vi "Main.vi"   [LabVIEW 2017]
uses:
  <vilib>/Platform/TimedLoop/XDataNode/timing_clust.ctl
  <vilib>/Platform/TimedLoop/XDataNode/nitl_modes.ctl
  <vilib>/Platform/TimedLoop/XDataNode/wakeup.ctl
  Controls/State.ctl
  <vilib>/platform/TimedLoop/XDataNode/XDataNode.xnode
  <vilib>/Platform/TimedLoop/XDataNode/XDNodeRunTimeDep.lvlib
types:
  T1 = typedef "State.ctl" = enum16{"Standby", "Initialize", "Pusher", "Live", "Norm Brake", "E-Stop"}
  T2 = typedef "XDNodeRunTimeDep.lvlib/timing_clust.ctl" = cluster{"Expected End [f-1]":u64, "Actual End [f-1]":u64, "Finished Late? [f-1]":bool, "Expected End [i-1]":u64, "Actual End [i-1]":u64, "Finished Late? [i-1]":bool, "Expected Start [i]":u64, "Actual Start [i]":u64, "Expected Start [f]":u64, "Actual Start [f]":u64, "Source Name":string, "Structure Name":string, "Period":i64, "Deadline":i64, "Offset":i64, "Start":i64, "Priority":i32, "Timeout":i32, "Mode":T3, "Wakeup Reason":T4, "Error":errorcluster, "Source Type":string, "Secondary Source Type":string, "Global End Time":u64, "Global Start Time":u64, "Frame Duration":u64, "Iteration Duration":u64, "Assigned CPU":i32, "I/O Scan Engine Mode":u32}
  T3 = typedef "XDNodeRunTimeDep.lvlib/nitl_modes.ctl" = enum32{"No Change", "Process missed periods, maintain original phase", "Discard missed periods, maintain original phase", "Process missed periods, ignore original phase", "Discard missed periods, ignore original phase"}
  T4 = typedef "XDNodeRunTimeDep.lvlib/wakeup.ctl" = enum32{"Normal", "Aborted", "Asynchronous wakeup", "Timing source error", "Timed loop error", "Timeout"}
  T5 = cluster{"X dtheta":sgl, "Y dtheta":sgl, "Z dtheta":sgl, "X accel":sgl, "Y accel":sgl, "Z accel":sgl, "Velocity":sgl, "IMU Fault":bool, "Time Since Last Tape":sgl, "Position":sgl}
  T6 = cluster{"Primary Battery 1 Voltage":sgl, "Primary Battery 2 Voltage":sgl, "Reserve Battery Voltage":sgl, "Primary Battery 1 Current":sgl, "Primary Battery 2 Current":sgl, "Reserve Battery Current":sgl, "Primary Battery 1 Temperature":sgl, "Primary Battery 2 Temperature":sgl, "Reserve Battery Temperature":sgl, "Primary Battery 1 Low":bool, "Primary Battery 2 Low":bool, "Reserve Battery Low":bool, "Primary Battery 1 Critical":bool, "Primary Battery 2 Critical":bool, "Reserve Battery Critical":bool, "Primary Battery 1 Hot":bool, "Primary Battery 2 Hot":bool, "Reserve Battery Hot":bool, "Frame Temperature":sgl, "Frame Hot":bool, "Ambient Pressure":sgl, "Tank Pressure":sgl, "Downstream Pressure":sgl, "Tank Pressue Low":bool, "Downstream Pressure Low":bool, "Tank Pressure Fault":bool, "Downstream Pressure Fault":bool, "IR 1 RAW":sgl, "IR 2 RAW":sgl, "IR Fault":bool, "Pusher Connected":bool, "Left Tape Count":u32, "Right Tape Count":u32, "Left Velocity":sgl, "Right Velocity":sgl, "Left LS Fault":bool, "Right LS Fault":bool, "Levitation Height":sgl, "Levitating?":bool, "PCS 1 Position":sgl, "PCS 2 Position":sgl, "PCS 3 Position":sgl, "PCS 4 Position":sgl, "FL Count":u8, "FR Count":u8, " BL Count":u8, "BR Count":u8}
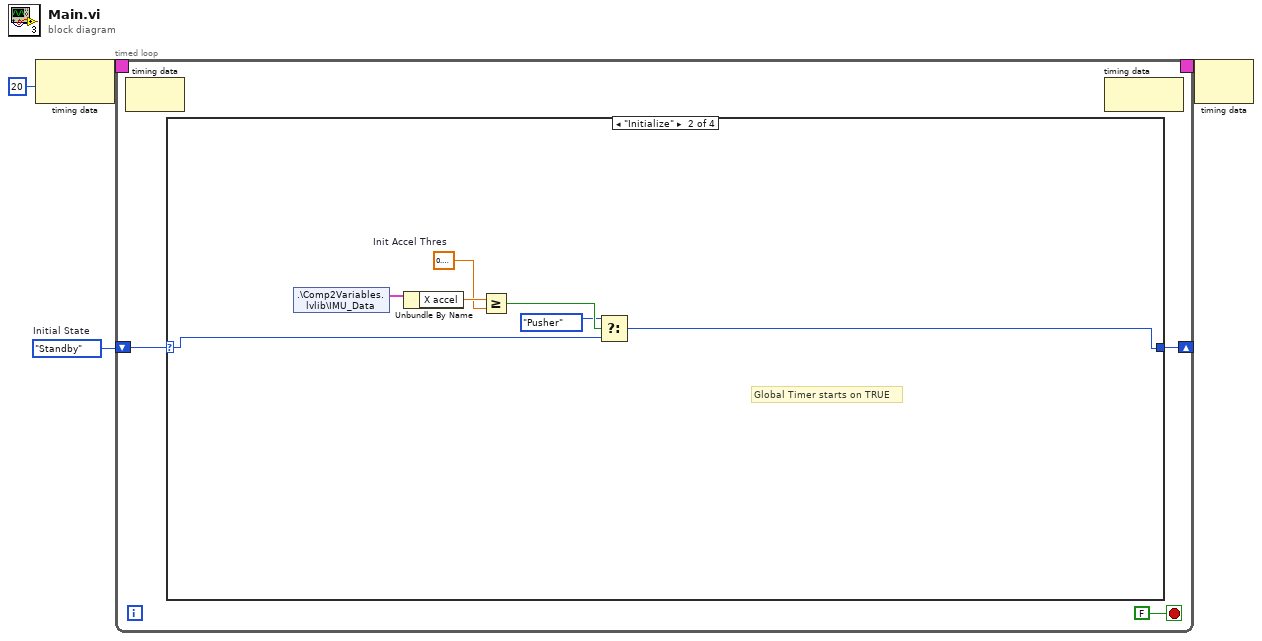
[diagram p0: block diagram]
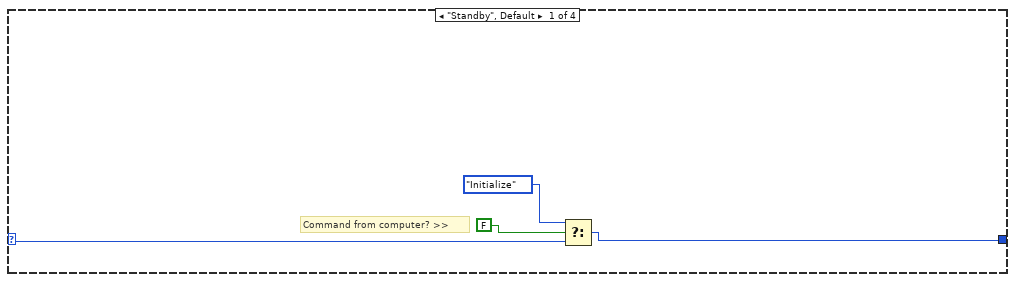
[diagram p2: hidden frame]
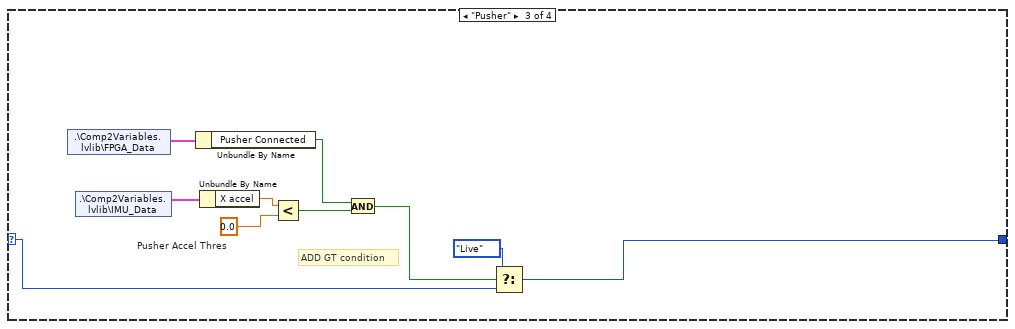
[diagram p3: hidden frame]
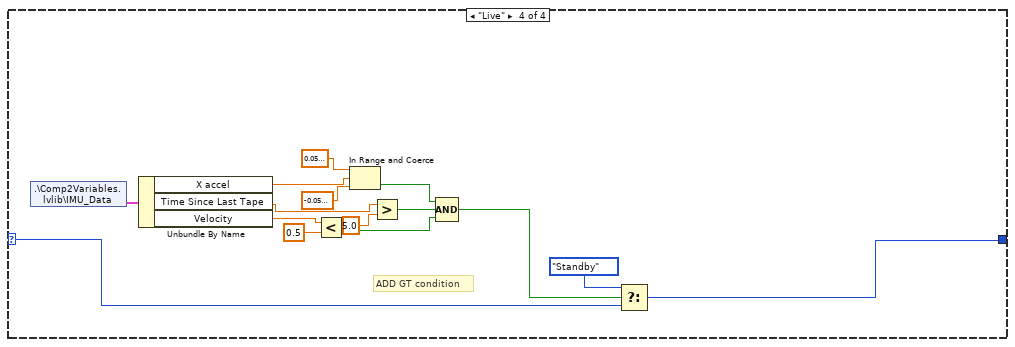
[diagram p4: hidden frame]
diagram:
  w1 = State."Standby"  # Initial State
  n1 = node-c288(i64 20 ("Period")) -> (w4:T2)
  n2 = timed-loop {
    timing: w4 -> [_]
    timing-out: [_] -> w3
    shift-right: [w5] -> _
    shift-left: w1 -> [w6]
    stop <- FALSE stop-if-true
    n3 = node-c288() -> ()  [unwired: 1 in, 1 out]
    n4 = case shown="\"Initialize\"" w6 {
      selector: w6 -> [w10 w13 w22 w31]
      tunnel: [w11 w12 w19 w30] -> w5
      frame "Standby", Default {
        # "Command from computer? >>"
        n5 = Select(t=State."Initialize" ("Initial State"), s=FALSE, f=w10) -> (s? t:f=w11:T1)
      }
      frame "Initialize" {
        w16 = sgl 0.2  # Init Accel Thres
        # "Global Timer starts on TRUE"
        n6 = shared-variable ".\\Comp2Variables.lvlib\\IMU_Data"() -> (w18:T5)  [unwired: 1 in, 1 out]
        n7 = Unbundle By Name(w18) -> ("X accel"=w17:sgl)
        n8 = Greater Or Equal?(x=w17, y=w16) -> (x >= y?=w15:bool)
        n9 = Select(t=State."Pusher", s=w15, f=w13) -> (s? t:f=w12:T1)
      }
      frame "Pusher" {
        w26 = sgl 0.0  # Pusher Accel Thres
        # "ADD GT condition"
        n10 = shared-variable ".\\Comp2Variables.lvlib\\FPGA_Data"() -> (w25:T6)  [unwired: 1 in, 1 out]
        n11 = shared-variable ".\\Comp2Variables.lvlib\\IMU_Data"() -> (w28:T5)  [unwired: 1 in, 1 out]
        n12 = Unbundle By Name(w25) -> ("Pusher Connected"=w24:bool)
        n13 = Unbundle By Name(w28) -> ("X accel"=w27:sgl)
        n14 = Less?(x=w27, y=w26) -> (x < y?=w23:bool)
        n15 = And(x=w24, y=w23) -> (x .and. y?=w21:bool)
        n16 = Select(t=State."Live" ("Initial State"), s=w21, f=w22) -> (s? t:f=w19:T1)
      }
      frame "Live" {
        # "ADD GT condition"
        n17 = shared-variable ".\\Comp2Variables.lvlib\\IMU_Data"() -> (w43:T5)  [unwired: 1 in, 1 out]
        n18 = Unbundle By Name(w43) -> ("X accel"=w42:sgl, "Time Since Last Tape"=w37:sgl, "Velocity"=w39:sgl)
        n19 = Less?(x=w39, y=sgl 0.5) -> (x < y?=w35:bool)
        n20 = In Range and Coerce(upper limit=sgl 0.05, x=w42, lower limit=sgl -0.05) -> (In Range?=w33:bool)  [unwired: 1 out]
        n21 = Greater?(x=w37, y=sgl 5.0) -> (0:w34:bool)
        n22 = Compound Arithmetic op=AND(w33, w34, w35) -> (w32:bool)
        n23 = Select(t=State."Standby" ("Initial State"), s=w32, f=w31) -> (s? t:f=w30:T1)
      }
    }
    n24 = node-c288() -> ()  [unwired: 1 in, 1 out]
  }
  n25 = node-c288(w3) -> ()  [unwired: 1 out]
